vi "Read field values.vi"(8 "error in (no error)":errorcluster, 11 "DbMeasurement in":refnum<class "DbMeasurement.lvclass">) -> (0 "error out":errorcluster, 1 "# pending insert":i32, 2 "# elements in queue":i32, 3 "DbMeasurement out":refnum<class "DbMeasurement.lvclass">, 4 "# pending remove":i32, 6 "Field Values Array":variant[](array[variant]))   [LabVIEW 2013, in "DbMeasurement.lvclass"]
doc: "This accessor gets the status of the field values queue."
uses:
  DbMeasurement.lvclass
  DbMeasurement.lvclass/DbMeasurement.ctl
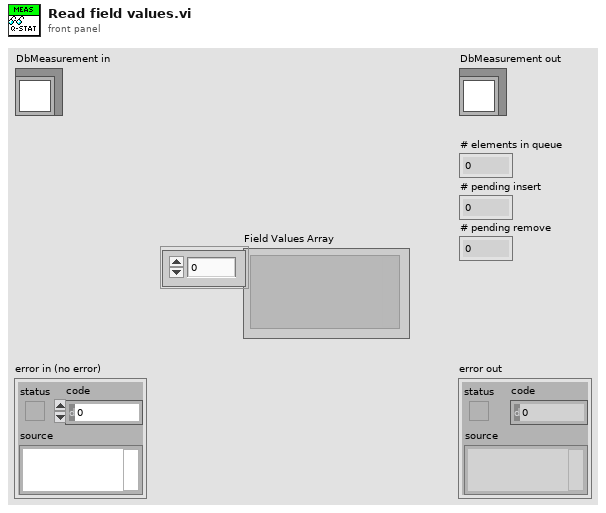
[diagram p1: front panel]
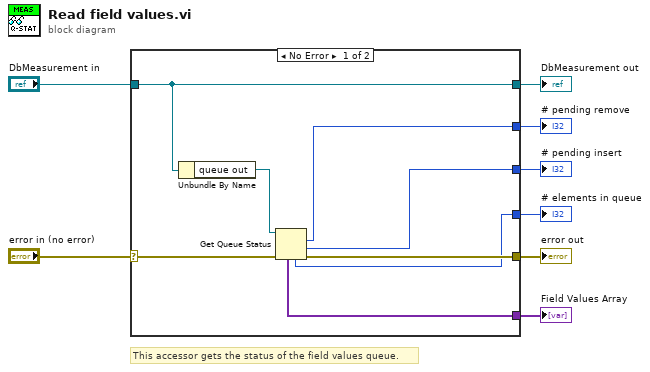
[diagram p0: block diagram]
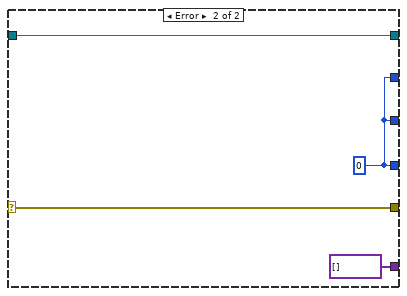
[diagram p2: hidden frame]
diagram:
  # "This accessor gets the status of the field values queue."
  n1 = case shown="No Error" "error in (no error)" {
    selector: "error in (no error)" -> [w15 w19]
    tunnel: [w14 w19] -> w7
    tunnel: [w16 w20] -> w5
    tunnel: "DbMeasurement in" -> [w16 w20]
    tunnel: [w12 variant[] [] ("elements")] -> w4
    tunnel: [w11 w17] -> w3
    tunnel: [w10 w17] -> w2
    tunnel: [w9 w17] -> w1
    frame No Error {
      n2 = Unbundle By Name(w16) -> ("queue out"=w13:refnum<queue>)
      n3 = Get Queue Status(queue=w13, error in (no error)=w15) -> (# pending remove=w11:i32, # pending insert=w9:i32, error out=w14:errorcluster, # elements in queue=w10:i32, elements=w12:variant[])  [unwired: 1 in, 3 out]
    }
    frame Error {
      w17 = 0 ("# elements in queue")
    }
  }
  "error out" <- w7
  "DbMeasurement out" <- w5
  "Field Values Array" <- w4
  "# pending remove" <- w3
  "# pending insert" <- w1
  "# elements in queue" <- w2
